vi "Wire To Unbundler Input Terminal.vi"(8 "error in (no error)":errorcluster, 10 "Terminal to be wired":refnum<vi>, 11 "Unbundler in":refnum<vi>) -> (0 "error out":errorcluster, 3 "Unbundler out":refnum<vi>)   [LabVIEW 2019, in "gRPC Template Creation Utility.lvlib"]
uses:
  gRPC Template Creation Utility.lvlib
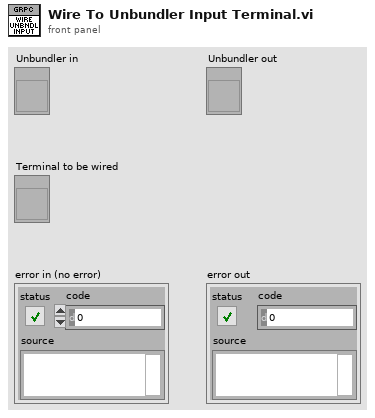
[diagram p1: front panel]
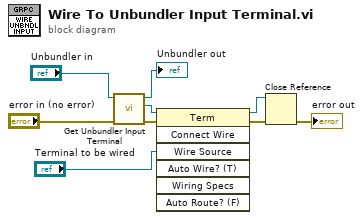
[diagram p0: block diagram]
diagram:
  n1 = call "Get Unbundler Input Terminal.vi"("error in (no error)"="error in (no error)", "Unbundler in"="Unbundler in") -> ("error out"=w5:errorcluster, "Unbundle Input Term Refnum"=w6:refnum<vi>, "Unbundler out"=→"Unbundler out":refnum<vi>)  [unwired: 7 in]
  n2 = invoke class="Term" method="Connect Wire"(reference=w6, error in=w5, "Wire Source"="Terminal to be wired") -> (reference out=w4:refnum<vi>, error out=w3:errorcluster)  [unwired: 4 in, 5 out]
  n3 = Close Reference(reference=w4, error in (no error)=w3) -> (error out=→"error out":errorcluster)
